vi "Format Error Message.vi"(4 "Code":i32, 6 "Error?":bool, 7 "Module":string, 8 "error in":errorcluster, 9 "Source":string, 10 "Message":string, 11 "Time Stamp":timestamp) -> (0 "error out":errorcluster, 1 "LabActor Error":T1, 2 "Formated error message":string)   [LabVIEW 2020]
uses:
  Template Module/LabActor Error.ctl
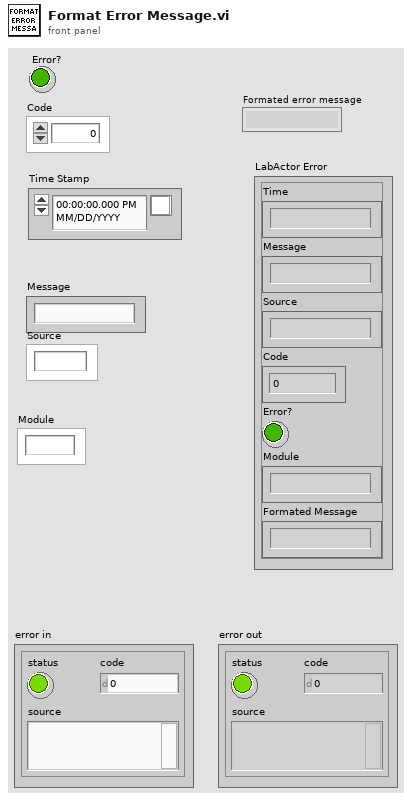
[diagram p1: front panel]
types:
  T1 = typedef "LabActor Error.ctl" = cluster{"Time":string, "Message":string, "Source":string, "Code":i32, "Error?":bool, "Module":string, "Formated Message":string}
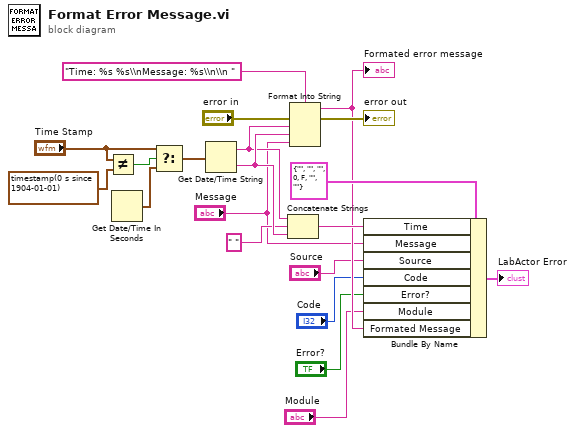
[diagram p0: block diagram]
diagram:
  n1 = Not Equal?(x="Time Stamp", y=timestamp(0 s since 1904-01-01) ("Time Stamp")) -> (x != y?=w19:bool)
  n2 = Get Date/Time In Seconds() -> (seconds since 1Jan1904=w17:timestamp)
  n3 = Select(t="Time Stamp", s=w19, f=w17) -> (s? t:f=w12:timestamp)
  n4 = Get Date/Time String(seconds (now)=w12) -> (date string=w14:string, time string=w16:string)  [unwired: 2 in]
  n5 = Concatenate Strings(w14, " " ("string"), w16) -> (w10:string)
  n6 = Format Into String(format string="Time: %s %s\\nMessage: %s\\n\\n ", error in="error in", w14, w16, "Message") -> (resulting string=w7:string, error out=→"error out":errorcluster)  [unwired: 1 in]
  "Formated error message" <- w7
  n7 = Bundle By Name(cluster=T1 {"Time"="", "Message"="", "Source"="", "Code"=0, "Error?"=FALSE, "Module"="", "Formated Message"=""} ("LabActor Error"), "Time"=w10, "Message"="Message", "Source"="Source", "Code"="Code", "Error?"="Error?", "Module"="Module", "Formated Message"=w7) -> (→"LabActor Error":T1)
